vi "Setup Statically-Linked subWorkers.vi"(8 "error in":errorcluster, 11 "gui in":refnum<class "gui.lvclass">) -> (0 "error out":errorcluster, 3 "gui out":refnum<class "gui.lvclass">)   [LabVIEW 2023, in "GUI.lvlib" / "gui.lvclass"]
doc: "This VI performs a setup of all the statically-linked subWorkers that belong to the Worker that owns this VI. This VI must be called <b>before</b> any statically-linked subWorkers are called."
uses:
  gui.lvclass
  gui.lvclass/gui.ctl
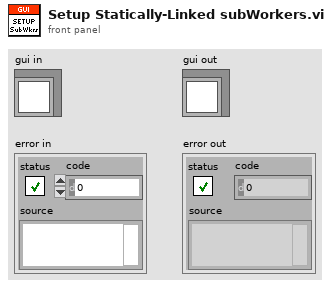
[diagram p1: front panel]
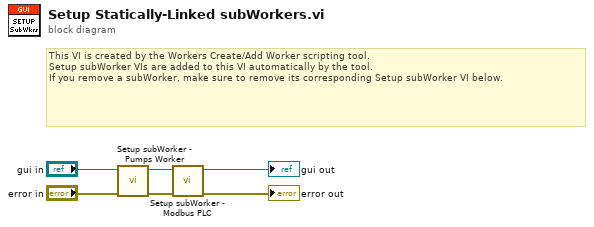
[diagram p0: block diagram]
diagram:
  # "This VI is created by the Workers Create/Add Worker scripting tool.\nSetup subWorker VIs are added to this VI automatically by the tool.\nIf you remove a subWorker, make sure to remove its corresponding Setup subWorker VI below."
  n1 = call "Setup subWorker - Pumps Worker.vi"("error in"="error in", "gui in"="gui in") -> ("error out"=w5:errorcluster, "gui out"=w3:refnum<class "gui.lvclass">)  [unwired: 8 in]
  n2 = call "Setup subWorker - Modbus PLC.vi"("error in"=w5, "gui in"=w3) -> ("error out"=→"error out":errorcluster, "gui out"=→"gui out":refnum<class "gui.lvclass">)  [unwired: 8 in]
